vi "VS_OpenProjectRef.vi"(0 "Engine Reference(in)":refnum<k7>, 1 "Condition Run?":bool, 2 "Requirement":string, 5 "Sequence File Ref(in)":refnum<k7>, 7 "VeriStand version info":T1, 9 "Project path":string="\"\"", 11 "error in":errorcluster, 12 "Step Group":i32(ring) items=["StepGroup_Setup", "StepGroup_Main", "StepGroup_Cleanup"], 13 "Step Index":i32) -> (4 "Engine reference(out)":refnum<k7>, 6 "Sequence File Ref(out)":refnum<k7>, 8 "VeriStand version info (out)":T1, 15 "error out":errorcluster)   [LabVIEW 2010]
doc: "This VI creates a TestStand step to open the reference to a VeriStand project"
uses:
  Ctls/dotNetAssemblyInfo.ctl
  Ctls/VSModuleTokens.ctl
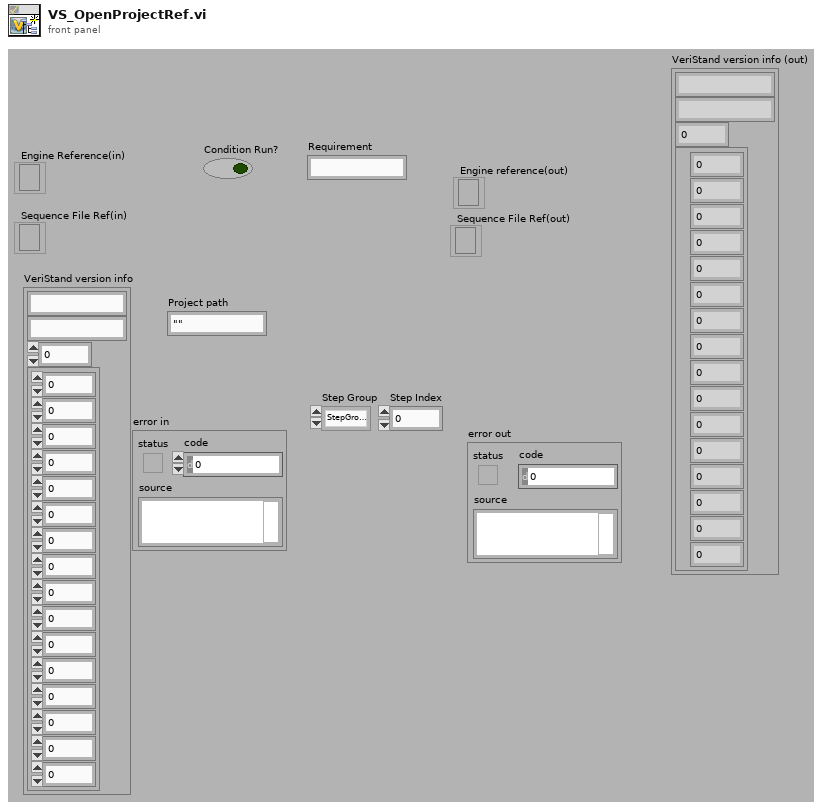
[diagram p1: front panel]
types:
  T1 = typedef "dotNetAssemblyInfo.ctl" = cluster{"VeriStand.exe Path":string, "Assembly":string, "Constructor Token":i32, "Module Token":T2}
  T2 = typedef "VSModuleTokens.ctl" = cluster{"GetIWorkspaceToken":i32, "GetIStimulusToken":i32, "GetIModelManagerToken":i32, "GetIProjectToken":i32, "RunProjectToken":i32, "CloseProjectToken":i32, "RunWorkspaceToken":i32, "StopWorkspaceToken":i32, "SetSingleChannelToken":i32, "SetMultipleParametersToken":i32, "RunStimulusToken":i32, "GetStimulusStateToken":i32, "Open WorkspaceToken":i32, "DeployToken":i32, "UndeployToken":i32, "QuitToken":i32}
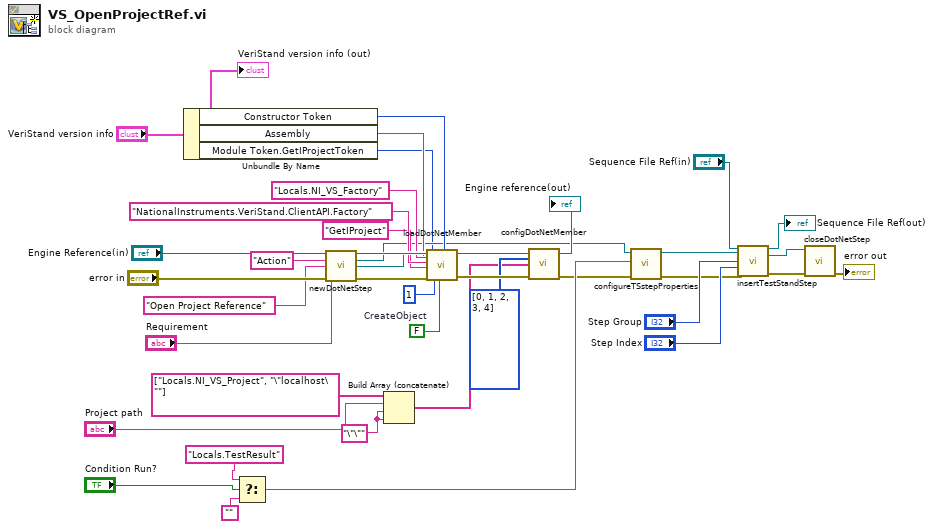
[diagram p0: block diagram]
diagram:
  w3 = "\"\""
  w23 = FALSE  # CreateObject
  n1 = Unbundle By Name("VeriStand version info") -> ("Constructor Token"=w17:i32, "Assembly"=w18:string, "Module Token.GetIProjectToken"=w6:i32)
  n2 = Select(t="Locals.TestResult", s="Condition Run?", f="") -> (s? t:f=w9:string)
  n3 = call "newDotNetStep.vi"("Engine reference"="Engine Reference(in)", "stepType"="Action", "Step Name"="Open Project Reference", "Requirement"="Requirement", "error in"="error in") -> ("Engine reference(out)"=→"Engine reference(out)":refnum<k7>, "NewStep (out)"=w11:refnum<k7>, "dotNetModule(out)"=w27:refnum<k7>, "error out"=w39:errorcluster)  [unwired: 7 in]
  n4 = Build Array (concatenate)(string[] ["Locals.NI_VS_Project", "\"localhost\""] ("Parameter Value array"), "Project path", w3, w3) -> (w4:string[])
  n5 = call "loadDotNetMember.vi"("dotNetModule"=w27, "Strong Assembly path"=w18, "ClassName"="NationalInstruments.VeriStand.ClientAPI.Factory", "MemberName"="GetIProject", "Member token"=w6, "error in(no error)"=w39, "ClassReference"="Locals.NI_VS_Factory", "Call Member?"=1 ("Call Memeber?"), "CreateObject"=w23, "Constructor Token"=w17) -> ("dotNetModule(out)"=w22:refnum<k7>, "error out"=w21:errorcluster)  [unwired: 8 in]
  n6 = call "configDotNetMember.vi"("dotNetModule"=w22, "Index array"=i32[] [0, 1, 2, 3, 4], "Parameter Value array"=w4, "error in (no error)"=w21) -> ("error out"=w8:errorcluster)  [unwired: 11 in]
  n7 = call "configureTSstepProperties.vi"("error in"=w8, "Precondition"=w9, "NewStep (in)"=w11) -> ("error out"=w7:errorcluster, "NewStep (out)"=w10:refnum<k7>)  [unwired: 7 in]
  n8 = call "insertTestStandStep.vi"("Sequence File Ref"="Sequence File Ref(in)", "Step to insert"=w10, "Step Group"="Step Group", "index"="Step Index", "error out"=w7) -> ("Sequence File Ref(out)"=→"Sequence File Ref(out)":refnum<k7>, "Step to insert (out)"=w38:refnum<k7>, "error out"=w36:errorcluster)  [unwired: 8 in]
  n9 = call "closeDotNetStep.vi"("error in"=w36, "NewStep"=w38) -> ("error out"=→"error out":errorcluster)  [unwired: 9 in]
  "VeriStand version info (out)" <- "VeriStand version info"
